vi "MultiListBoxSort.vi"() -> ()   [LabVIEW 2011]
panel:
  in  "Multicolumn Listbox":i32(listbox)
  in  "stop":bool
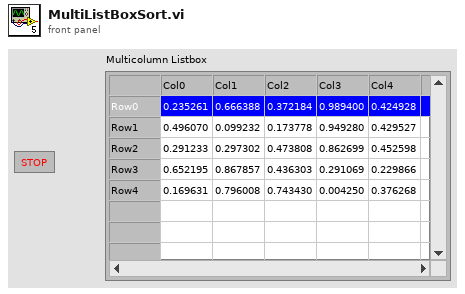
[diagram p1: front panel]
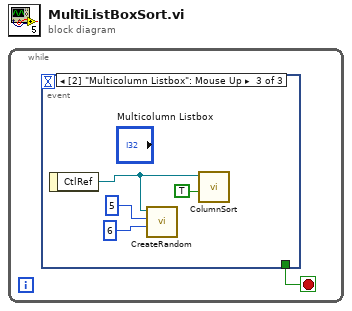
[diagram p0: block diagram]
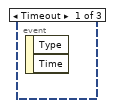
[diagram p2: hidden frame]
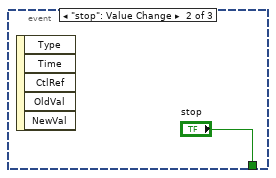
[diagram p3: hidden frame]
diagram:
  n1 = while {
    stop <- w1 stop-if-true
    n2 = event shown="[2] \"Multicolumn Listbox\": Mouse Up" {
      selector: _ -> [_ _ _]
      dyn-events: _ -> [_ _ _]
      timeout: _ -> [_ _ _]
      tunnel: [_ "stop" _] -> w1
      event Timeout {
        n3 = event-data() -> ()  [unwired: 1 in, 2 out]
      }
      event "stop": Value Change {
        n4 = event-data() -> ()  [unwired: 1 in, 5 out]
      }
      event "Multicolumn Listbox": Mouse Up {
        n5 = event-data() -> ("CtlRef"=w5:refnum<vi>)  [unwired: 1 in]
        n6 = call "CreateRandom.vi"("Col"=6, "Row"=5, "MCListbox Refnum"=w5) -> ()  [unwired: 8 in, 1 out]
        n7 = call "ColumnSort.vi"("Desend"=TRUE, "MCListbox Refnum"=w5) -> ()  [unwired: 9 in, 1 out]
      }
    }
  }
